vi "LogDialog.vi"(8 "Error In":errorcluster, 10 "Executable Configuration":T4, 11 "Log Configuration In":T5) -> (0 "Error Out":errorcluster, 2 "Cancelled?":bool, 3 "Log Configuration Out":T5)   [LabVIEW 2012]
uses:
  LogConfiguration.ctl
  LogStartConfiguration.ctl
  LogStartTriggerType.ctl
  LogDigitalIOTriggerEdge.ctl
  LogRolloverConfiguration.ctl
  LogRolloverTriggerType.ctl
  LogStopConfiguration.ctl
  LogStopTriggerType.ctl
  ExecutableConfiguration.ctl
  libs/LV-Utilities/LV-Utilities.lvlib
panel:
  in  "Stop Digital IO Edge":enum16{"Rising", "Falling"}(ring)
  in  "Stop Digital IO Line":u8=1 min=1 max=14 step=1
  in  "Stop File Size (MB)":u32=256
  in  "Stop Timer (sec)":dbl format="%<%H:%M:%S>t"
  in  "Stop Trigger Type":T1(ring)
  in  "Start Digital IO Edge":enum16{"Rising", "Falling"}(ring)
  in  "Start Digital IO Line":u8=1 min=1 max=14 step=1
  in  "Start Timer (sec)":dbl format="%<%H:%M:%S>t"
  in  "Start Trigger Type":T2(ring)
  in  "Rollover Digital IO Edge":enum16{"Rising", "Falling"}(ring)
  in  "Rollover Digital IO Line":u8=1 min=1 max=14 step=1
  in  "Rollover File Size (MB)":u32=256
  in  "Rollover Timer (sec)":dbl format="%<%H:%M:%S>t"
  in  "Rollover Trigger Type":T3(ring)
  in  "CANCEL":bool
  in  "DONE":bool
  # "STOP"
  # "Digital IO Edge"
  # "Digital IO Line"
  # "File Size"
  # "Timer"
  # "Type"
  # "START"
  # "Digital IO Edge"
  # "Digital IO Line"
  # "Timer"
  # "Type"
  # "ROLLOVER"
  # "Digital IO Edge"
  # "Digital IO Line"
  # "File Size"
  # "Timer"
  # "Type"
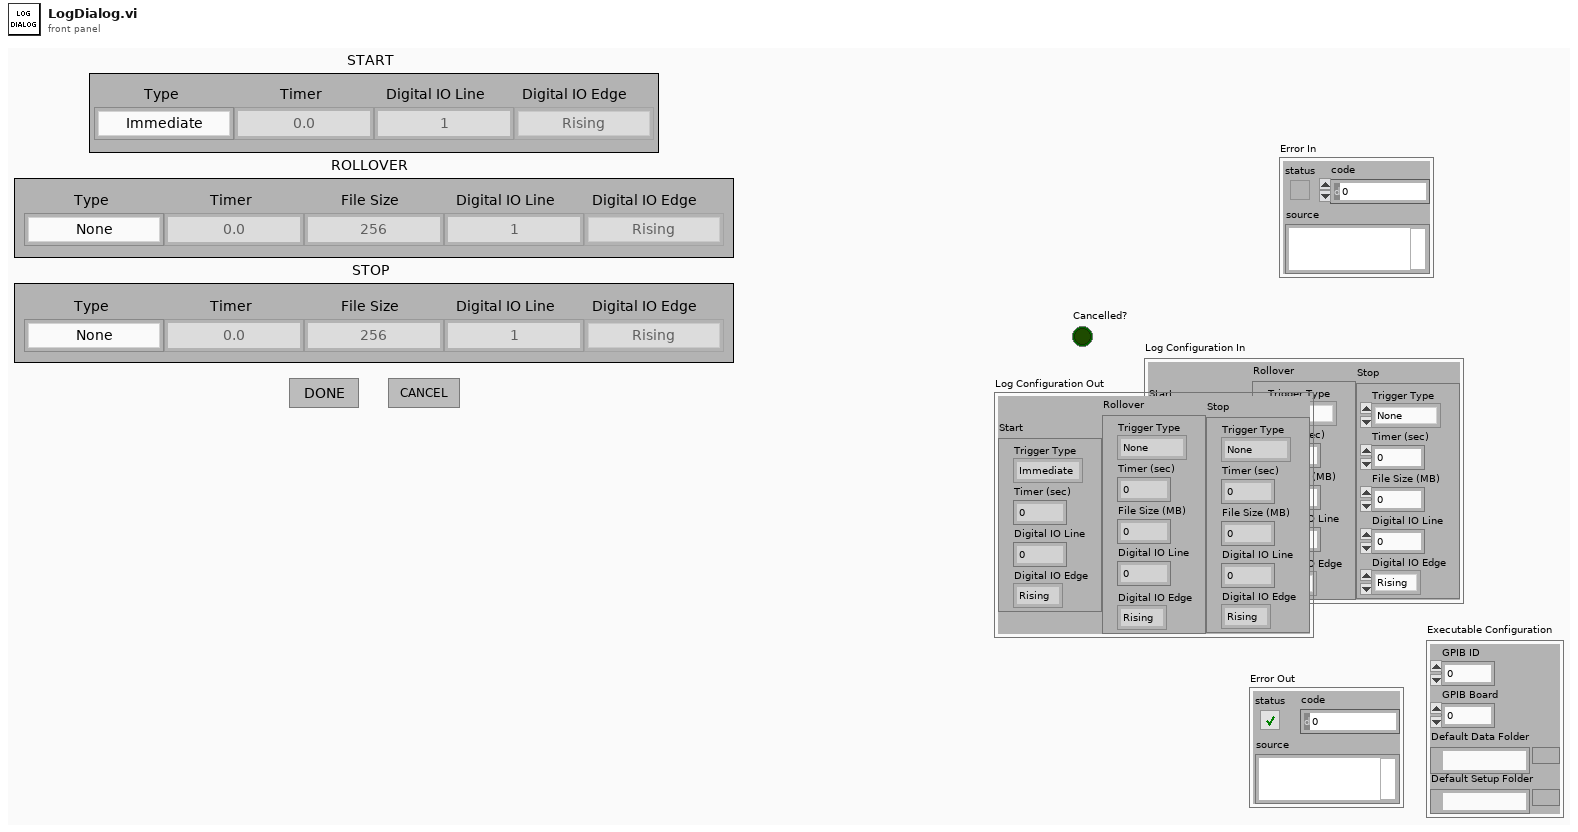
[diagram p1: front panel]
types:
  T1 = enum16{"None", "User", "Timer", "File Size", "Digital IO"}
  T2 = enum16{"Immediate", "User", "Timer", "Digital IO"}
  T3 = enum16{"None", "Timer", "File Size", "Digital IO"}
  T4 = typedef "ExecutableConfiguration.ctl" = cluster{"GPIB ID":u8, "GPIB Board":u8, "Default Data Folder":path, "Default Setup Folder":path}
  T5 = typedef "LogConfiguration.ctl" = cluster{"Start":T6, "Rollover":T9, "Stop":T11}
  T6 = typedef "LogStartConfiguration.ctl" = cluster{"Trigger Type":T7, "Timer (sec)":dbl, "Digital IO Line":u8, "Digital IO Edge":T8}
  T7 = typedef "LogStartTriggerType.ctl" = enum16{"Immediate", "User", "Timer", "Digital IO"}
  T8 = typedef "LogDigitalIOTriggerEdge.ctl" = enum16{"Rising", "Falling"}
  T9 = typedef "LogRolloverConfiguration.ctl" = cluster{"Trigger Type":T10, "Timer (sec)":dbl, "File Size (MB)":u32, "Digital IO Line":u8, "Digital IO Edge":T8}
  T10 = typedef "LogRolloverTriggerType.ctl" = enum16{"None", "Timer", "File Size", "Digital IO"}
  T11 = typedef "LogStopConfiguration.ctl" = cluster{"Trigger Type":T12, "Timer (sec)":dbl, "File Size (MB)":u32, "Digital IO Line":u8, "Digital IO Edge":T8}
  T12 = typedef "LogStopTriggerType.ctl" = enum16{"None", "User", "Timer", "File Size", "Digital IO"}
  T13 = enum8{"Enabled", "Disabled", "Disabled and Grayed Out"}
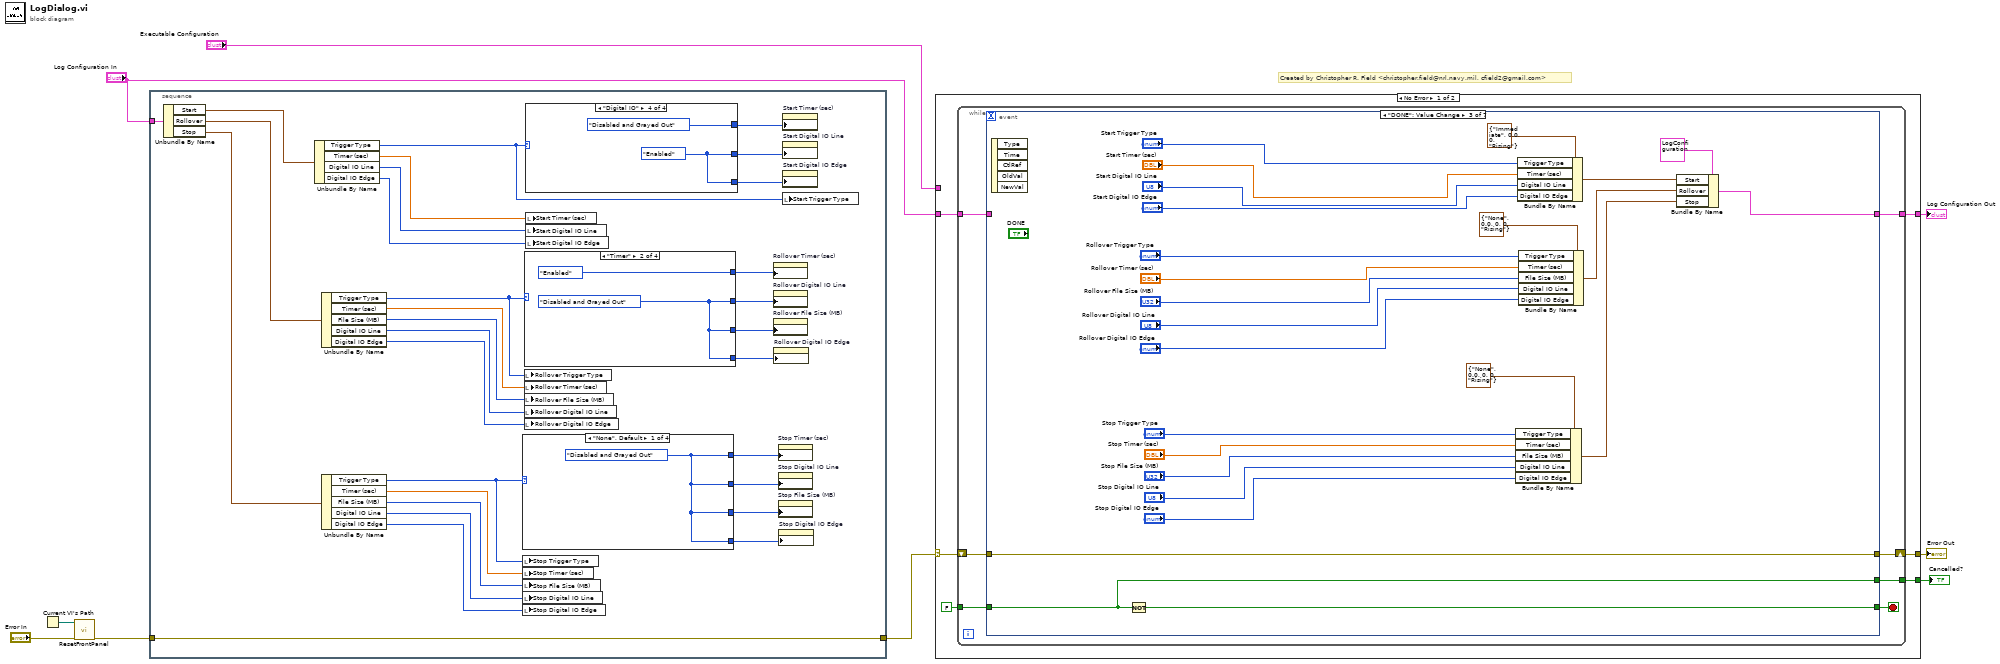
[diagram p0: block diagram]
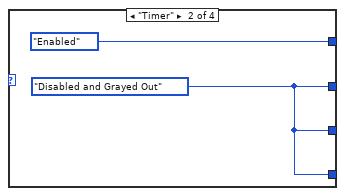
[diagram p2: hidden frame]
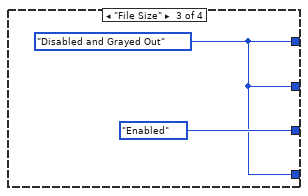
[diagram p3: hidden frame]
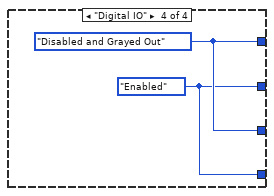
[diagram p4: hidden frame]
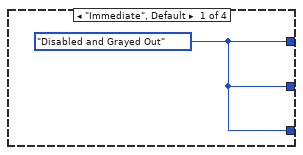
[diagram p5: hidden frame]
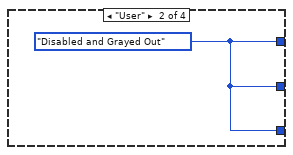
[diagram p6: hidden frame]
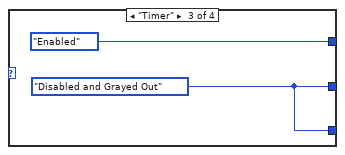
[diagram p7: hidden frame]
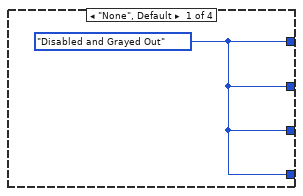
[diagram p8: hidden frame]
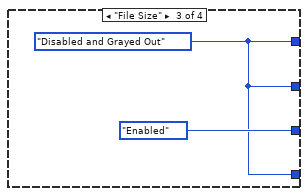
[diagram p9: hidden frame]
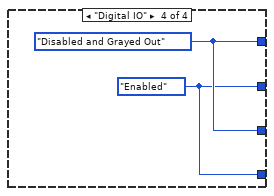
[diagram p10: hidden frame]
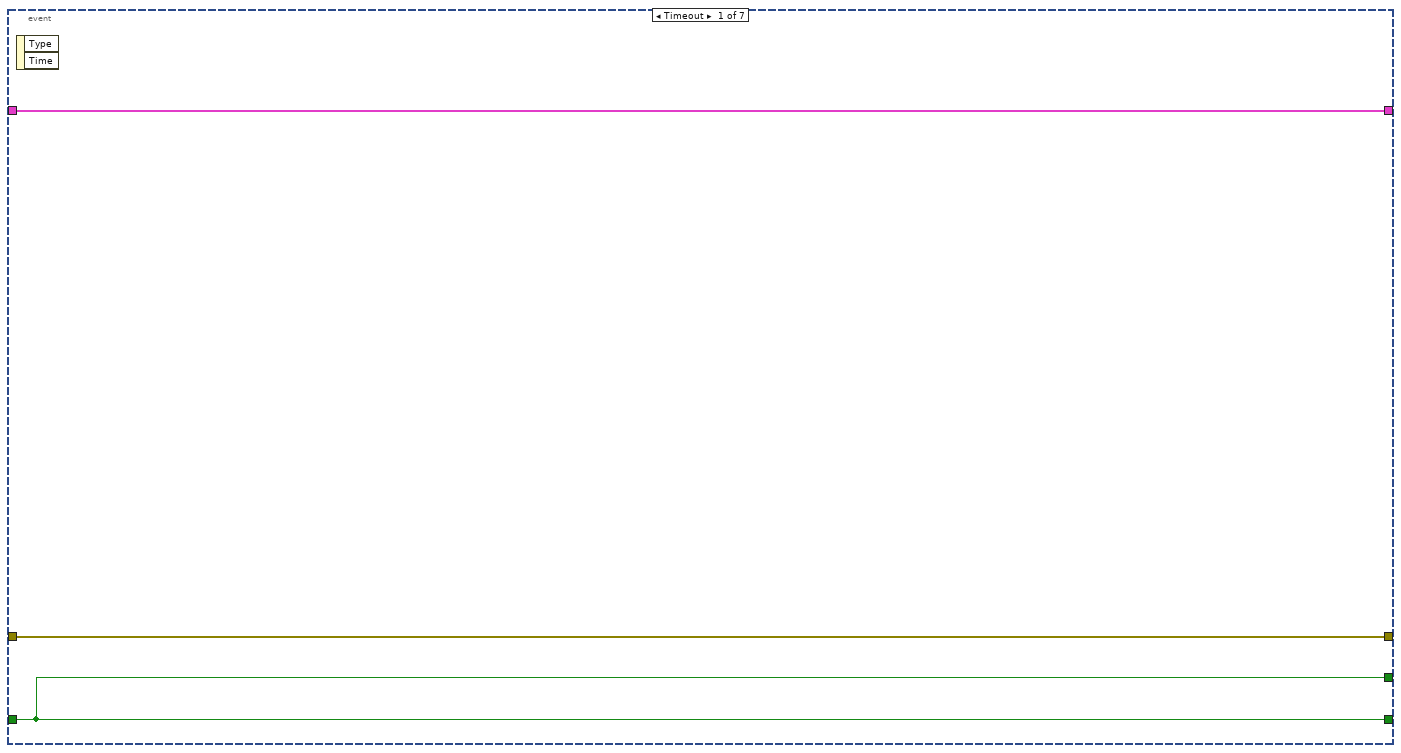
[diagram p11: hidden frame]
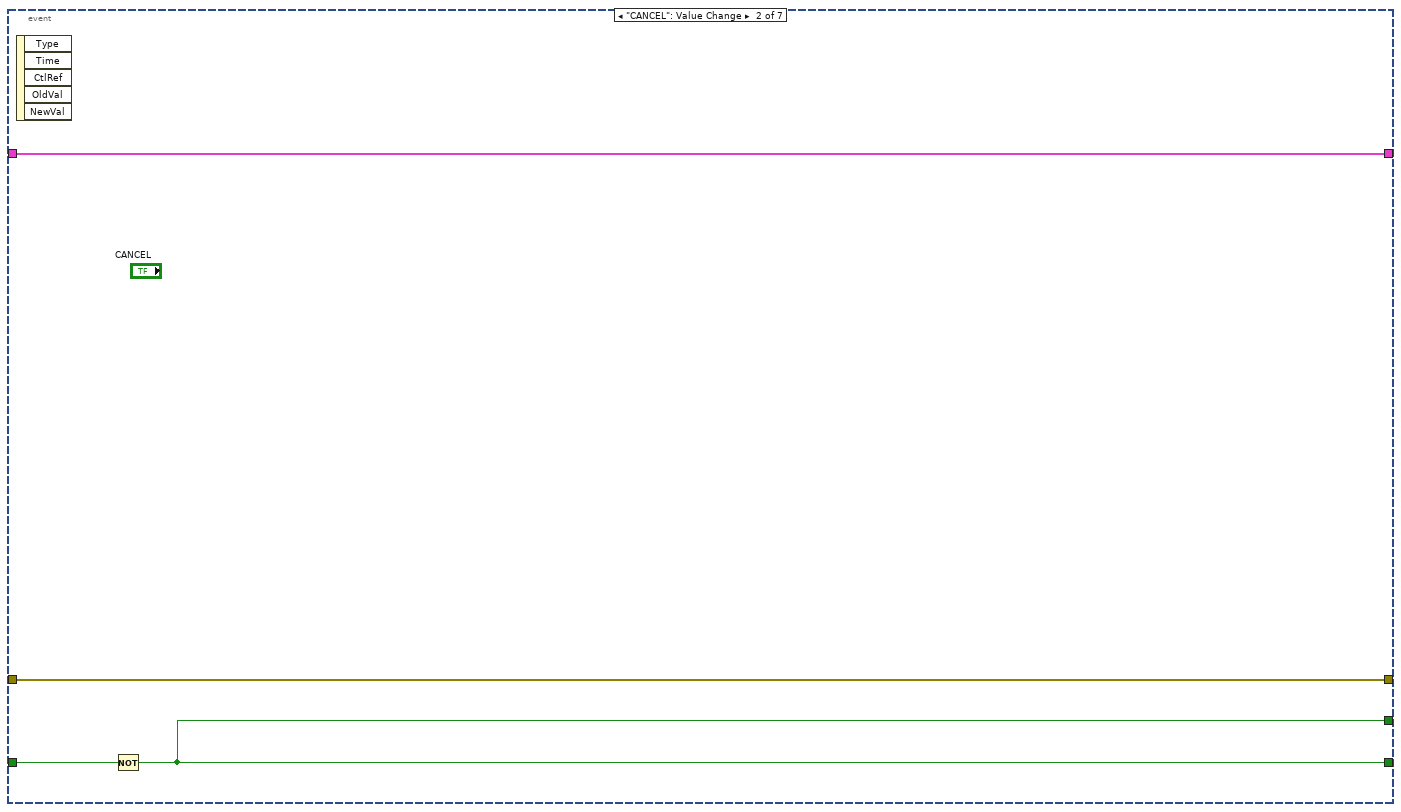
[diagram p12: hidden frame]
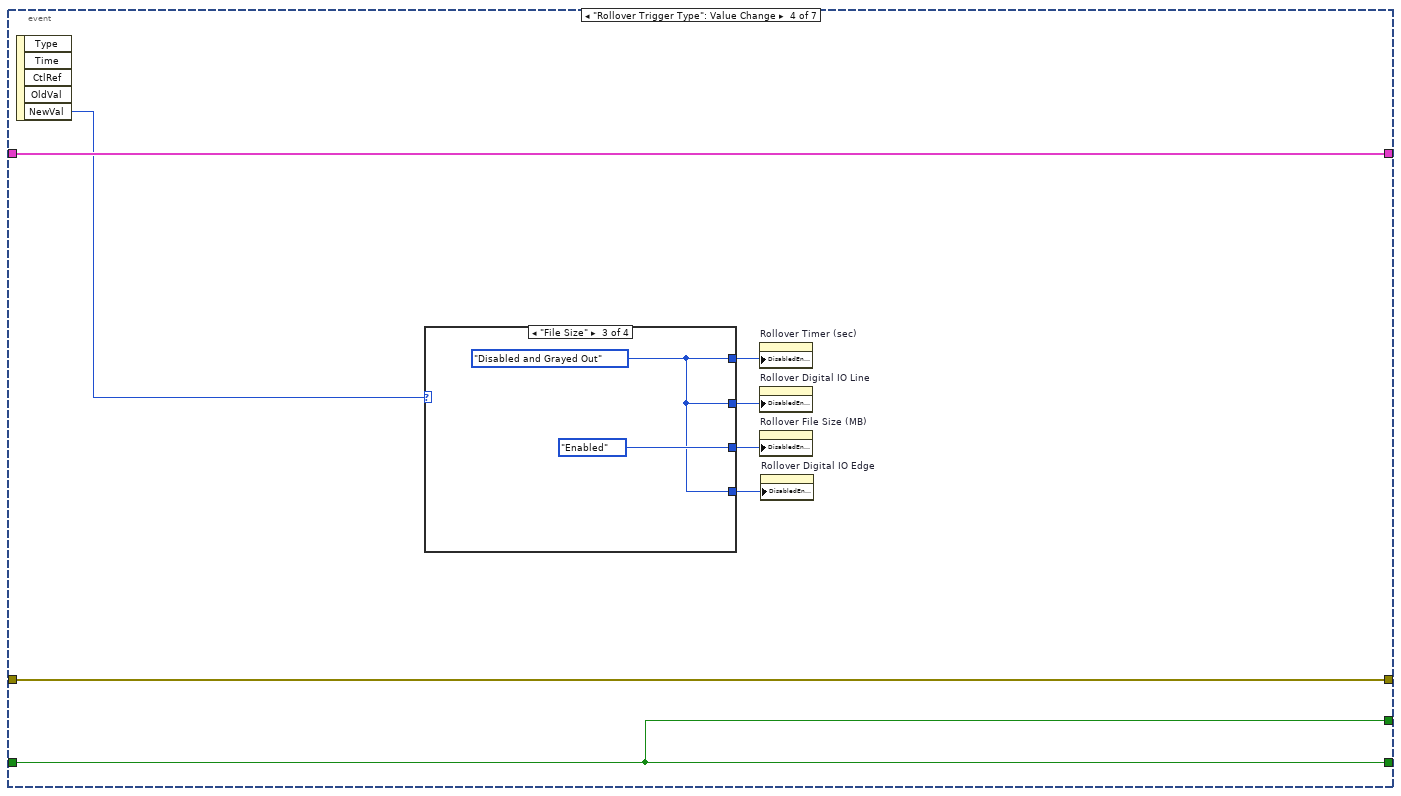
[diagram p13: hidden frame]
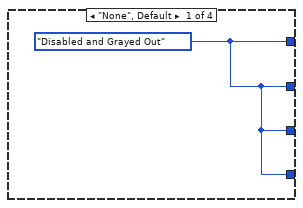
[diagram p14: hidden frame]
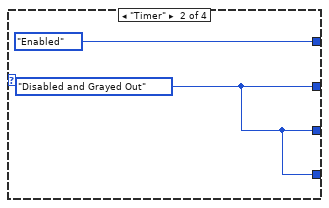
[diagram p15: hidden frame]
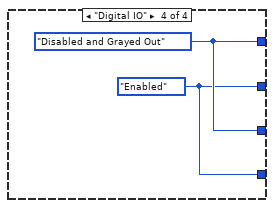
[diagram p16: hidden frame]
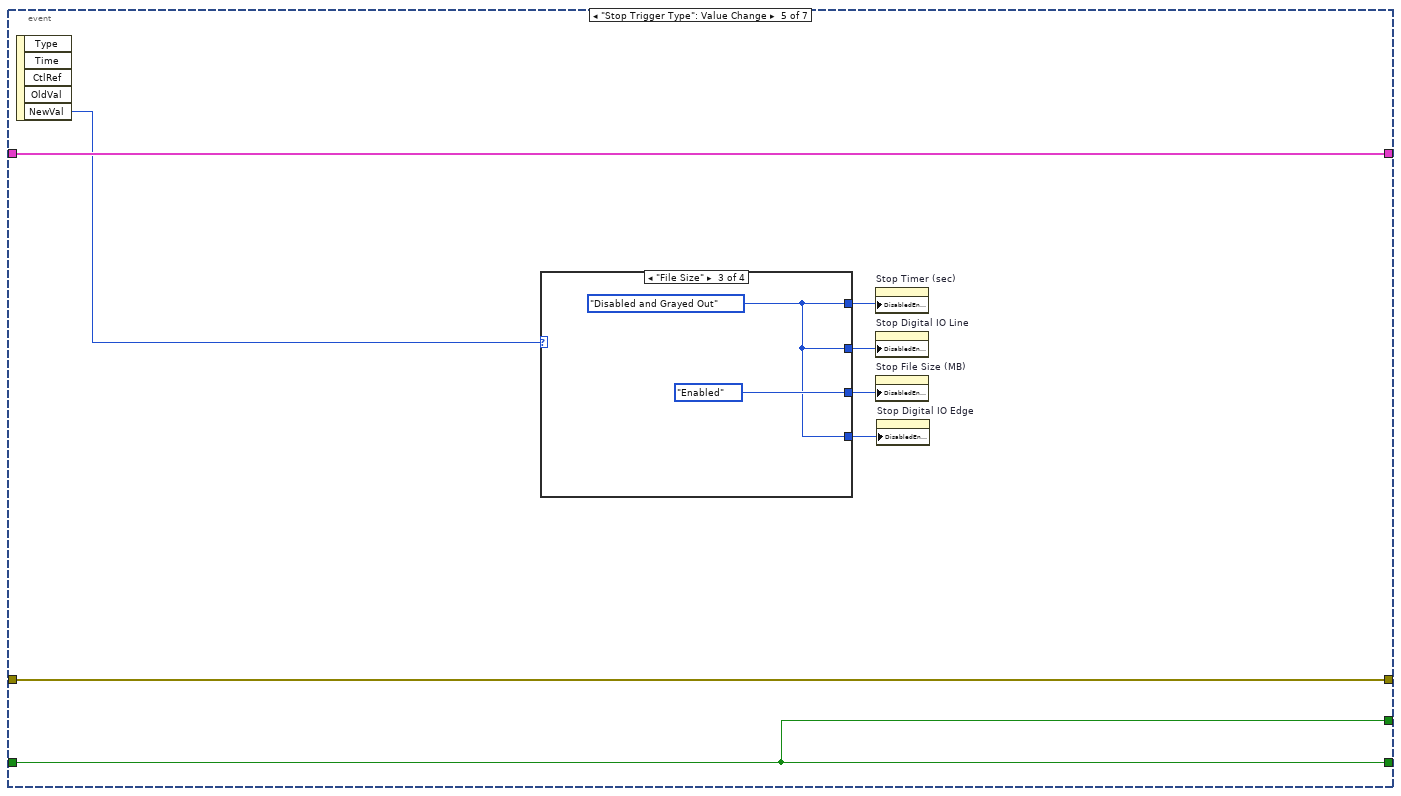
[diagram p17: hidden frame]
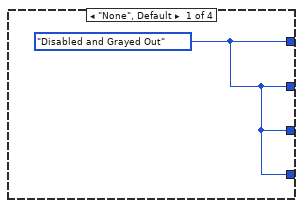
[diagram p18: hidden frame]
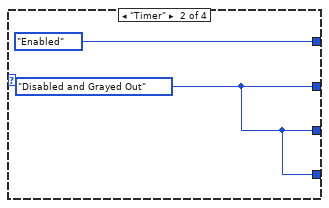
[diagram p19: hidden frame]
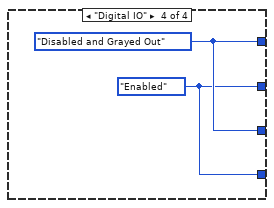
[diagram p20: hidden frame]
diagram:
  # "Created by Christopher R. Field <christopher.field@nrl.navy.mil, cfield2@gmail.com>"
  n1 = Current VI's Path() -> (path=w9:path)
  n2 = call "ResetFrontPanel.vi"("Error In"="Error In", "VI Path"=w9) -> ("Error Out"=w5:errorcluster)  [unwired: 9 in]
  n3 = stacked-sequence {
    tunnel: w5 -> [w39]
    tunnel: [w39] -> w4
    tunnel: "Log Configuration In" -> [w35]
    frame #0 {
      n4 = Unbundle By Name(w35) -> ("Start"=w27:T6, "Rollover"=w34:T9, "Stop"=w26:T11)
      n5 = Unbundle By Name(w27) -> ("Trigger Type"=w10:T7, "Timer (sec)"=w18:dbl, "Digital IO Line"=w17:u8, "Digital IO Edge"=w16:T8)
      n6 = Unbundle By Name(w34) -> ("Trigger Type"=w32:T10, "Timer (sec)"=w31:dbl, "File Size (MB)"=w30:u32, "Digital IO Line"=w29:u8, "Digital IO Edge"=w28:T8)
      n7 = Unbundle By Name(w26) -> ("Trigger Type"=w15:T12, "Timer (sec)"=w14:dbl, "File Size (MB)"=w13:u32, "Digital IO Line"=w12:u8, "Digital IO Edge"=w11:T8)
      n8 = case shown="\"None\", Default" w15 {
        tunnel: [w40 T13."Enabled" ("Disabled") w43 w46] -> w25
        tunnel: [w40 w41 w43 w45] -> w24
        tunnel: [w40 w41 T13."Enabled" ("Disabled") w46] -> w23
        tunnel: [w40 w41 w43 w45] -> w22
        frame "None", Default {
          w40 = T13."Disabled and Grayed Out" ("Disabled")
        }
        frame "Timer" {
          w41 = T13."Disabled and Grayed Out" ("Disabled")
        }
        frame "File Size" {
          w43 = T13."Disabled and Grayed Out" ("Disabled")
        }
        frame "Digital IO" {
          w45 = T13."Enabled" ("Disabled")
          w46 = T13."Disabled and Grayed Out" ("Disabled")
        }
      }
      n9 = local write "Stop Trigger Type"(w15) -> ()
      n10 = local write "Stop Timer (sec)"(w14) -> ()
      n11 = local write "Stop File Size (MB)"(w13) -> ()
      n12 = local write "Stop Digital IO Line"(w12) -> ()
      n13 = local write "Stop Digital IO Edge"(w11) -> ()
      n14 = case shown="\"Timer\"" w32 {
        tunnel: [w53 T13."Enabled" ("Disabled") w56 w59] -> w38
        tunnel: [w53 w54 w56 w58] -> w37
        tunnel: [w53 w54 T13."Enabled" ("Disabled") w59] -> w36
        tunnel: [w53 w54 w56 w58] -> w33
        frame "None", Default {
          w53 = T13."Disabled and Grayed Out" ("Disabled")
        }
        frame "Timer" {
          w54 = T13."Disabled and Grayed Out" ("Disabled")
        }
        frame "File Size" {
          w56 = T13."Disabled and Grayed Out" ("Disabled")
        }
        frame "Digital IO" {
          w58 = T13."Enabled" ("Disabled")
          w59 = T13."Disabled and Grayed Out" ("Disabled")
        }
      }
      n15 = local write "Rollover Trigger Type"(w32) -> ()
      n16 = local write "Rollover Timer (sec)"(w31) -> ()
      n17 = local write "Rollover File Size (MB)"(w30) -> ()
      n18 = local write "Rollover Digital IO Line"(w29) -> ()
      n19 = local write "Rollover Digital IO Edge"(w28) -> ()
      n20 = case shown="\"Digital IO\"" w10 {
        tunnel: [w47 w48 T13."Enabled" ("Disabled") T13."Disabled and Grayed Out" ("Disabled")] -> w21
        tunnel: [w47 w48 w49 w51] -> w20
        tunnel: [w47 w48 w49 w51] -> w19
        frame "Immediate", Default {
          w47 = T13."Disabled and Grayed Out" ("Disabled")
        }
        frame "User" {
          w48 = T13."Disabled and Grayed Out" ("Disabled")
        }
        frame "Timer" {
          w49 = T13."Disabled and Grayed Out" ("Disabled")
        }
        frame "Digital IO" {
          w51 = T13."Enabled" ("Disabled")
        }
      }
      n21 = local write "Start Timer (sec)"(w18) -> ()
      n22 = local write "Start Digital IO Line"(w17) -> ()
      n23 = local write "Start Digital IO Edge"(w16) -> ()
      n24 = property on="Rollover Timer (sec)" class="DigNum (strict)"("DisabledEnum"=w38) -> ()  [unwired: 2 in, 2 out]
      n25 = property on="Rollover Digital IO Line" class="DigNum (strict)"("DisabledEnum"=w37) -> ()  [unwired: 2 in, 2 out]
      n26 = property on="Rollover File Size (MB)" class="DigNum (strict)"("DisabledEnum"=w36) -> ()  [unwired: 2 in, 2 out]
      n27 = property on="Rollover Digital IO Edge" class="Enum (strict)"("DisabledEnum"=w33) -> ()  [unwired: 2 in, 2 out]
      n28 = property on="Stop Timer (sec)" class="DigNum (strict)"("DisabledEnum"=w25) -> ()  [unwired: 2 in, 2 out]
      n29 = property on="Stop Digital IO Line" class="DigNum (strict)"("DisabledEnum"=w24) -> ()  [unwired: 2 in, 2 out]
      n30 = property on="Stop File Size (MB)" class="DigNum (strict)"("DisabledEnum"=w23) -> ()  [unwired: 2 in, 2 out]
      n31 = property on="Stop Digital IO Edge" class="Enum (strict)"("DisabledEnum"=w22) -> ()  [unwired: 2 in, 2 out]
      n32 = property on="Start Timer (sec)" class="DigNum (strict)"("DisabledEnum"=w21) -> ()  [unwired: 2 in, 2 out]
      n33 = property on="Start Digital IO Line" class="DigNum (strict)"("DisabledEnum"=w20) -> ()  [unwired: 2 in, 2 out]
      n34 = property on="Start Digital IO Edge" class="Enum (strict)"("DisabledEnum"=w19) -> ()  [unwired: 2 in, 2 out]
      n35 = local write "Start Trigger Type"(w10) -> ()
    }
  }
  n36 = case shown="No Error" w4 {
    selector: w4 -> [w64 w154]
    tunnel: [w63 w154] -> w7
    tunnel: [w62 FALSE] -> w6
    tunnel: "Log Configuration In" -> [w61 w152]
    tunnel: [w60 w152] -> w2
    tunnel: "Executable Configuration" -> [_ _]
    frame No Error {
      n37 = while {
        tunnel: FALSE -> [w72]
        shift-right: [w69] -> w63
        shift-left: w64 -> [w70]
        tunnel: [w68] -> w62
        tunnel: w61 -> [w67]
        tunnel: [w66] -> w60
        stop <- w71 stop-if-true
        n38 = event shown="[2] \"DONE\": Value Change" {
          selector: _ -> [_ _ _ _ _ _ _]
          dyn-events: _ -> [_ _ _ _ _ _ _]
          timeout: _ -> [_ _ _ _ _ _ _]
          tunnel: w72 -> [w74 w77 w102 w110 w125 w135 w150]
          tunnel: [w74 w76 w103 w110 w125 w135 w149] -> w71
          tunnel: w70 -> [w75 w78 w104 w111 w126 w136 w151]
          tunnel: [w75 w78 w104 w111 w126 w136 w151] -> w69
          tunnel: [w74 w76 w102 w110 w125 w135 w149] -> w68
          tunnel: w67 -> [w73 w79 _ w112 w127 w138 w148]
          tunnel: [w73 w79 w81 w112 w127 w138 w148] -> w66
          event Timeout {
            n39 = event-data() -> ()  [unwired: 1 in, 2 out]
          }
          event "CANCEL": Value Change {
            n40 = event-data() -> ()  [unwired: 1 in, 5 out]
            n41 = Not(x=w77) -> (.not. x?=w76:bool)
          }
          event "DONE": Value Change {
            n42 = event-data() -> ()  [unwired: 1 in, 5 out]
            n43 = Not(x=w102) -> (.not. x?=w103:bool)
            n44 = Bundle By Name(cluster=T11 {"Trigger Type"=enum."None", "Timer (sec)"=0.0, "File Size (MB)"=0, "Digital IO Line"=0, "Digital IO Edge"=enum."Rising"} ("Log Stop Configuration"), "Trigger Type"="Stop Trigger Type", "Timer (sec)"="Stop Timer (sec)", "File Size (MB)"="Stop File Size (MB)", "Digital IO Line"="Stop Digital IO Line", "Digital IO Edge"="Stop Digital IO Edge") -> (w82:T11)
            n45 = Bundle By Name(cluster=T6 {"Trigger Type"=enum."Immediate", "Timer (sec)"=0.0, "Digital IO Line"=0, "Digital IO Edge"=enum."Rising"} ("Log Start Configuration"), "Trigger Type"="Start Trigger Type", "Timer (sec)"="Start Timer (sec)", "Digital IO Line"="Start Digital IO Line", "Digital IO Edge"="Start Digital IO Edge") -> (w84:T6)
            n46 = Bundle By Name(cluster=T9 {"Trigger Type"=enum."None", "Timer (sec)"=0.0, "File Size (MB)"=0, "Digital IO Line"=0, "Digital IO Edge"=enum."Rising"} ("Log Rollover Configuration"), "Trigger Type"="Rollover Trigger Type", "Timer (sec)"="Rollover Timer (sec)", "File Size (MB)"="Rollover File Size (MB)", "Digital IO Line"="Rollover Digital IO Line", "Digital IO Edge"="Rollover Digital IO Edge") -> (w83:T9)
            n47 = Bundle By Name(cluster=T5 {"Start"={"Trigger Type"=enum."Immediate", "Timer (sec)"=0.0, "Digital IO Line"=0, "Digital IO Edge"=enum."Rising"}, "Rollover"={"Trigger Type"=enum."None", "Timer (sec)"=0.0, "File Size (MB)"=0, "Digital IO Line"=0, "Digital IO Edge"=enum."Rising"}, "Stop"={"Trigger Type"=enum."None", "Timer (sec)"=0.0, "File Size (MB)"=0, "Digital IO Line"=0, "Digital IO Edge"=enum."Rising"}} ("Log Configuration"), "Start"=w84, "Rollover"=w83, "Stop"=w82) -> (w81:T5)
          }
          event "Rollover Trigger Type": Value Change {
            n48 = event-data() -> ("NewVal"=w109:T3)  [unwired: 1 in, 4 out]
            n49 = case shown="\"File Size\"" w109 {
              tunnel: [w113 T13."Enabled" ("Disabled") w116 w119] -> w108
              tunnel: [w113 w114 w116 w118] -> w107
              tunnel: [w113 w114 T13."Enabled" ("Disabled") w119] -> w106
              tunnel: [w113 w114 w116 w118] -> w105
              frame "None", Default {
                w113 = T13."Disabled and Grayed Out" ("Disabled")
              }
              frame "Timer" {
                w114 = T13."Disabled and Grayed Out" ("Disabled")
              }
              frame "File Size" {
                w116 = T13."Disabled and Grayed Out" ("Disabled")
              }
              frame "Digital IO" {
                w118 = T13."Enabled" ("Disabled")
                w119 = T13."Disabled and Grayed Out" ("Disabled")
              }
            }
            n50 = property on="Rollover Timer (sec)" class="DigNum (strict)"("DisabledEnum"=w108) -> ()  [unwired: 2 in, 2 out]
            n51 = property on="Rollover Digital IO Line" class="DigNum (strict)"("DisabledEnum"=w107) -> ()  [unwired: 2 in, 2 out]
            n52 = property on="Rollover File Size (MB)" class="DigNum (strict)"("DisabledEnum"=w106) -> ()  [unwired: 2 in, 2 out]
            n53 = property on="Rollover Digital IO Edge" class="Enum (strict)"("DisabledEnum"=w105) -> ()  [unwired: 2 in, 2 out]
          }
          event "Stop Trigger Type": Value Change {
            n54 = event-data() -> ("NewVal"=w120:T1)  [unwired: 1 in, 4 out]
            n55 = case shown="\"File Size\"" w120 {
              tunnel: [w128 T13."Enabled" ("Disabled") w131 w134] -> w124
              tunnel: [w128 w129 w131 w133] -> w123
              tunnel: [w128 w129 T13."Enabled" ("Disabled") w134] -> w122
              tunnel: [w128 w129 w131 w133] -> w121
              frame "None", Default {
                w128 = T13."Disabled and Grayed Out" ("Disabled")
              }
              frame "Timer" {
                w129 = T13."Disabled and Grayed Out" ("Disabled")
              }
              frame "File Size" {
                w131 = T13."Disabled and Grayed Out" ("Disabled")
              }
              frame "Digital IO" {
                w133 = T13."Enabled" ("Disabled")
                w134 = T13."Disabled and Grayed Out" ("Disabled")
              }
            }
            n56 = property on="Stop Timer (sec)" class="DigNum (strict)"("DisabledEnum"=w124) -> ()  [unwired: 2 in, 2 out]
            n57 = property on="Stop Digital IO Line" class="DigNum (strict)"("DisabledEnum"=w123) -> ()  [unwired: 2 in, 2 out]
            n58 = property on="Stop File Size (MB)" class="DigNum (strict)"("DisabledEnum"=w122) -> ()  [unwired: 2 in, 2 out]
            n59 = property on="Stop Digital IO Edge" class="Enum (strict)"("DisabledEnum"=w121) -> ()  [unwired: 2 in, 2 out]
          }
          event "Start Trigger Type": Value Change {
            n60 = event-data() -> ("NewVal"=w137:T2)  [unwired: 1 in, 4 out]
            n61 = case shown="\"Digital IO\"" w137 {
              tunnel: [w142 w143 T13."Enabled" ("Disabled") T13."Disabled and Grayed Out" ("Disabled")] -> w141
              tunnel: [w142 w143 w144 w146] -> w140
              tunnel: [w142 w143 w144 w146] -> w139
              frame "Immediate", Default {
                w142 = T13."Disabled and Grayed Out" ("Disabled")
              }
              frame "User" {
                w143 = T13."Disabled and Grayed Out" ("Disabled")
              }
              frame "Timer" {
                w144 = T13."Disabled and Grayed Out" ("Disabled")
              }
              frame "Digital IO" {
                w146 = T13."Enabled" ("Disabled")
              }
            }
            n62 = property on="Start Timer (sec)" class="DigNum (strict)"("DisabledEnum"=w141) -> ()  [unwired: 2 in, 2 out]
            n63 = property on="Start Digital IO Line" class="DigNum (strict)"("DisabledEnum"=w140) -> ()  [unwired: 2 in, 2 out]
            n64 = property on="Start Digital IO Edge" class="Enum (strict)"("DisabledEnum"=w139) -> ()  [unwired: 2 in, 2 out]
          }
          event Panel Close? {
            n65 = event-data() -> ()  [unwired: 1 in, 3 out]
            n66 = Not(x=w150) -> (.not. x?=w149:bool)
            n67 = event-data("Discard?"=w149) -> ()  [unwired: 1 in, 1 out]
          }
        }
      }
    }
    frame Error {
    }
  }
  "Error Out" <- w7
  "Cancelled?" <- w6
  "Log Configuration Out" <- w2
